vi "get8elementsHORIBLE.vi"(0 "Array":dbl[](array[numeric])) -> (20 "Numeric":dbl, 21 "Numeric 2":dbl, 22 "Numeric 3":dbl, 23 "Numeric 4":dbl, 24 "Numeric 5":dbl, 25 "Numeric 6":dbl, 26 "Numeric 7":dbl, 27 "Numeric 8":dbl)   [LabVIEW 2015]
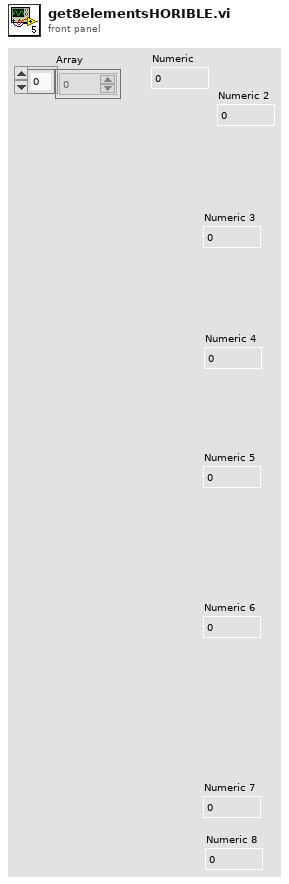
[diagram p1: front panel]
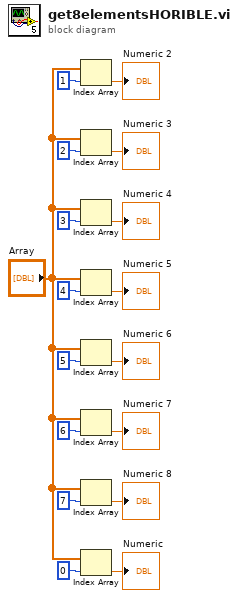
[diagram p0: block diagram]
diagram:
  n1 = Index Array(array="Array", index=1) -> (element=→"Numeric 2":dbl)
  n2 = Index Array(array="Array", index=2) -> (element=→"Numeric 3":dbl)
  n3 = Index Array(array="Array", index=3) -> (element=→"Numeric 4":dbl)
  n4 = Index Array(array="Array", index=4) -> (element=→"Numeric 5":dbl)
  n5 = Index Array(array="Array", index=5) -> (element=→"Numeric 6":dbl)
  n6 = Index Array(array="Array", index=6) -> (element=→"Numeric 7":dbl)
  n7 = Index Array(array="Array", index=7) -> (element=→"Numeric 8":dbl)
  n8 = Index Array(array="Array", index=0) -> (element=→"Numeric":dbl)
